vi "NewAccessor.vi"(11 "Object":T1) -> ()   [LabVIEW 2018, in "LVClassByRef.lvlib"]
uses:
  <resource>/Framework/Providers/LVClassByRef/LVClassByRef.lvlib
  <resource>/Framework/Providers/API/ItemRef.ctl
  <resource>/Framework/Providers/LVClassByRef/Accessor Options.ctl
panel:
  in  "Property":bool=TRUE
  in  "Cancel":bool
  in  "Dynamic":bool
  in  "Setter":bool
  in  "Getter":bool=TRUE
  in  "Create":bool
  in  "Location":string(tree)
  in  "Class Item":string(tree)
  # "Type"
  # "Select location to create:"
  # "Accessor Type(s):"
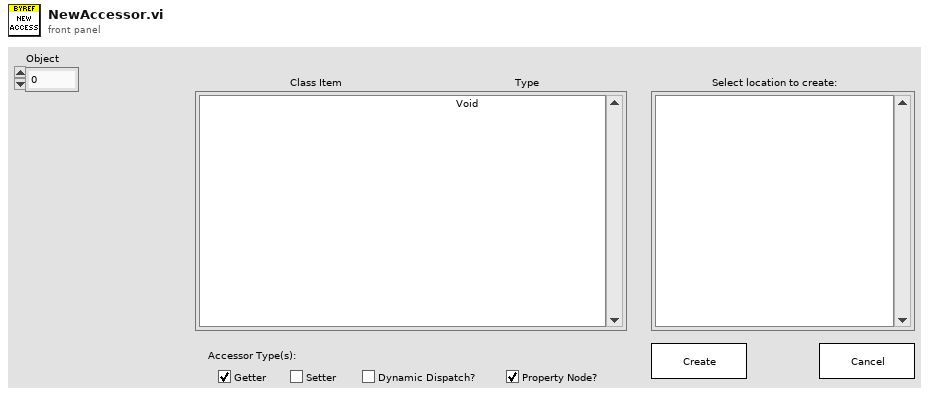
[diagram p1: front panel]
types:
  T1 = typedef "ItemRef.ctl" = u64
  T2 = typedef "LVClassByRef.lvlib/Folder Item.ctl" = cluster{"Tree":T3, "Item":refnum<vi>}
  T3 = typedef "LVClassByRef.lvlib/Tree Item.ctl" = cluster{"Name":string, "Depth":i32, "Parent":i32}
  T4 = typedef "LVClassByRef.lvlib/Type Item.ctl" = cluster{"Tree":T3, "Value":variant, "Children":i32[], "Selectable?":bool, "Type":T5}
  T5 = typedef "NI_Data Type.lvlib/Data Type.ctl" = enum8{"Invalid Type", "Void", "I8", "I16", "I32", "I64", "U8", "U16", "U32", "U64", "Single Float", "Double Float", "Extended Float", "Single Complex", "Double Complex", "Extended Complex", "Enum U8", "Enum U16", "Enum U32", "Enum U64", "Single Float With Unit", "Double Float With Unit", "Extended Float With Unit", "Single Complex with Unit", "Double Complex with Unit", "Extended Complex with Unit", "Boolean", "String", "Path", "Picture", "Tag", "Array", "Cluster", "Variant", "LV Variant", "Waveform", "Timestamp", "Digital Waveform", "Digital Data", "ExpressData", "Refnum", "External Data", "VI", "Poly VI", "LabVIEW Class Instance", "Fixed Point"}
  T6 = typedef "LVClassByRef.lvlib/Accessor Options.ctl" = cluster{"Item Path":string, "Project Path":string, "Getter":bool, "Setter":bool, "Dynamic":bool, "Property":bool}
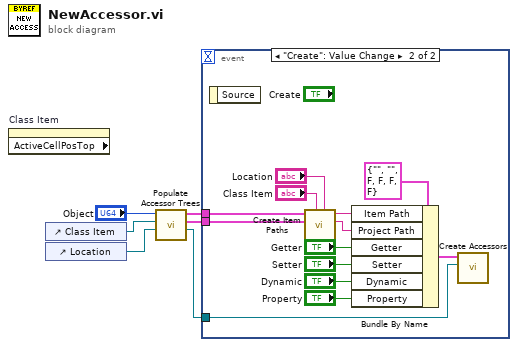
[diagram p0: block diagram]
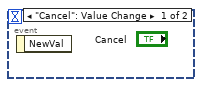
[diagram p2: hidden frame]
diagram:
  n1 = property on="Class Item" class="Tree (strict)" props=["ActiveCellPosTop"]() -> ()  [unwired: 2 in, 3 out]
  n2 = control-ref of="Class Item"() -> (w5:refnum<vi>)
  n3 = control-ref of="Location"() -> (w4:refnum<vi>)
  n4 = call <resource>:"Populate Accessor Trees.vi"("Folder Tree Ref"=w4, "Class Item Tree Ref"=w5, "Class"="Object") -> ("LVClassLibrary"=w1:refnum<vi>, "Folder Tree"=w2:T2[], "Type Tree"=w3:T4[])  [unwired: 6 in]
  n5 = event shown="[1] \"Create\": Value Change" {
    selector: _ -> [_ _]
    dyn-events: _ -> [_ _]
    timeout: _ -> [_ _]
    tunnel: w3 -> [_ w19]
    tunnel: w2 -> [_ w18]
    tunnel: w1 -> [_ w9]
    event "Cancel": Value Change {
      n6 = event-data() -> ()  [unwired: 1 in, 1 out]
    }
    event "Create": Value Change {
      n7 = event-data() -> ()  [unwired: 1 in, 1 out]
      n8 = call <resource>:"Create Item Paths.vi"("Folder Row"="Location", "Type Row"="Class Item", "Folder Tree"=w18, "Type Tree"=w19) -> ("Project Path"=w15:string, "Type Path"=w16:string)  [unwired: 6 in]
      n9 = Bundle By Name(cluster=T6 {"Item Path"="", "Project Path"="", "Getter"=FALSE, "Setter"=FALSE, "Dynamic"=FALSE, "Property"=FALSE} ("Accessor Options"), "Item Path"=w16, "Project Path"=w15, "Getter"="Getter", "Setter"="Setter", "Dynamic"="Dynamic", "Property"="Property") -> (w10:T6)
      n10 = call <resource>:"Create Accessors.vi"("LVClassLibrary"=w9, "Accessor Options"=w10) -> ()  [unwired: 10 in]
    }
  }
